vi "Update name of exp.vi"(8 "error in (no error)":errorcluster, 9 "Exp name":string, 10 "Exp #":i32, 11 "Control-Client in":refnum<class "Control-Client.lvclass">) -> (0 "error out":errorcluster, 3 "Control-Client out":refnum<class "Control-Client.lvclass">)   [LabVIEW 2018]
uses:
  Control-Client.lvclass
  Control-Client.lvclass/Control-Client.ctl
  methods/Read Group #.vi
  Experiments/Experiments_group.lvclass
  Experiments/Experiment.lvclass
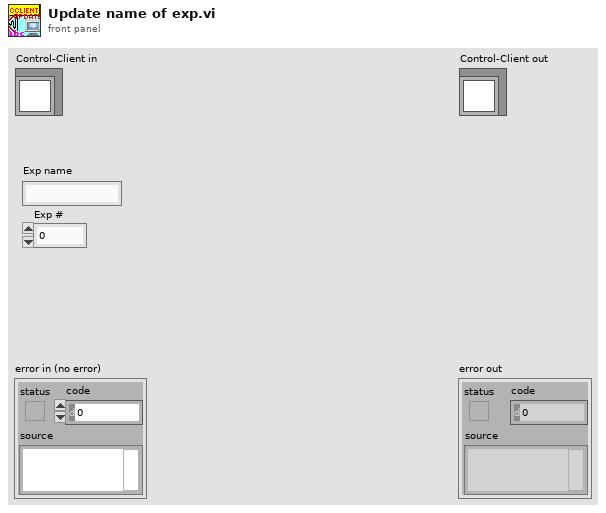
[diagram p1: front panel]
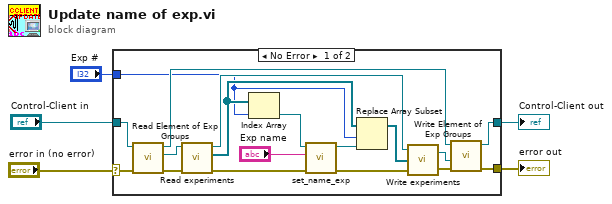
[diagram p0: block diagram]
diagram:
  n1 = case shown="No Error" "error in (no error)" {
    selector: "error in (no error)" -> [w7 w25]
    tunnel: [w10 w25] -> w4
    tunnel: [w11 w24] -> w2
    tunnel: "Control-Client in" -> [w23 w24]
    tunnel: "Exp #" -> [w6 _]
    frame No Error {
      n2 = call "Read Element of Exp Groups.vi"("error in (no error)"=w7, "Control-Client in"=w23) -> ("error out"=w22:errorcluster, "Experiments_group.lvclass"=w21:refnum<class "Experiments_group.lvclass">, "Control-Client out"=w12:refnum<class "Control-Client.lvclass">)  [unwired: 7 in]
      n3 = call "Read experiments.vi"("error in (no error)"=w22, "Experiments_group.lvclass in"=w21) -> ("error out"=w16:errorcluster, "Experiments"=w18:refnum<class "Experiment.lvclass">[], "Experiments_group.lvclass out"=w14:refnum<class "Experiments_group.lvclass">)  [unwired: 6 in]
      n4 = Index Array(array=w18, index=w6) -> (element=w20:refnum<class "Experiment.lvclass">)
      n5 = call "set_name_exp.vi"("error in (no error)"=w16, "Exp name"="Exp name", "Experiment.lvclass in"=w20) -> ("error out"=w8:errorcluster, "Experiment.lvclass out"=w17:refnum<class "Experiment.lvclass">)  [unwired: 7 in]
      n6 = Replace Array Subset(array=w18, new element=w17, index=w6) -> (w15:refnum<class "Experiment.lvclass">[])
      n7 = call-dynamic "Write experiments.vi"("error in (no error)"=w8, "Experiments"=w15, "Experiments_group.lvclass in"=w14) -> ("error out"=w9:errorcluster, "Experiments_group.lvclass out"=w13:refnum<class "Experiments_group.lvclass">)
      n8 = call "Write Element of Exp Groups.vi"("error in (no error)"=w9, "Experiments_group.lvclass"=w13, "Control-Client in"=w12) -> ("error out"=w10:errorcluster, "Control-Client out"=w11:refnum<class "Control-Client.lvclass">)  [unwired: 7 in]
    }
    frame Error {
    }
  }
  "error out" <- w4
  "Control-Client out" <- w2
